vi "General-GetMultValue.vi"(1 "Ultimo Intervalo":dbl, 2 "Primer Intervalo":dbl, 3 "Tiempo Final":dbl, 4 "t":dbl) -> (0 "Out":dbl)   [LabVIEW 2010]
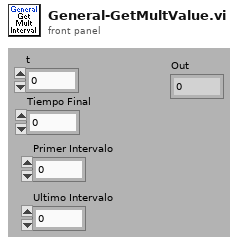
[diagram p1: front panel]
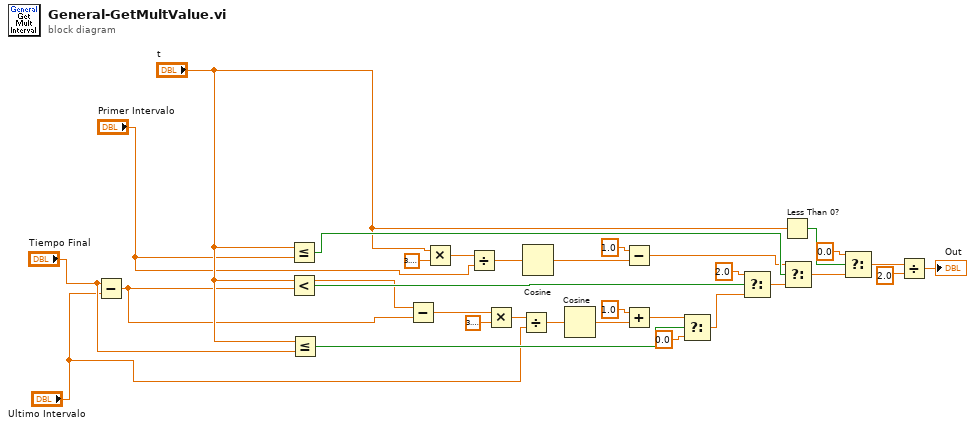
[diagram p0: block diagram]
diagram:
  n1 = Subtract(x="Tiempo Final", y="Ultimo Intervalo") -> (x-y=w3:dbl)
  n2 = Less Or Equal?(x="t", y="Primer Intervalo") -> (x <= y?=w29:bool)
  n3 = Less?(x="t", y=w3) -> (x < y?=w17:bool)
  n4 = Less Or Equal?(x="t", y="Tiempo Final") -> (x <= y?=w10:bool)
  n5 = Subtract(x="t", y=w3) -> (x-y=w14:dbl)
  n6 = Multiply(x="t", y=3.141592653589793) -> (x*y=w28:dbl)
  n7 = Divide(x=w28, y="Primer Intervalo") -> (x/y=w26:dbl)
  n8 = Multiply(x=w14, y=3.141592653589793) -> (x*y=w22:dbl)
  n9 = Divide(x=w22, y="Ultimo Intervalo") -> (x/y=w20:dbl)
  n10 = Cosine(x=w26) -> (cos(x)=w24:dbl)
  n11 = Cosine(x=w20) -> (cos(x)=w18:dbl)
  n12 = Subtract(x=1.0, y=w24) -> (x-y=w13:dbl)
  n13 = Add(x=1.0, y=w18) -> (x+y=w9:dbl)
  n14 = Select(t=w9, s=w10, f=0.0) -> (s? t:f=w7:dbl)
  n15 = Select(t=2.0, s=w17, f=w7) -> (s? t:f=w15:dbl)
  n16 = Less Than 0?(x="t") -> (x < 0?=w31:bool)
  n17 = Select(t=w13, s=w29, f=w15) -> (s? t:f=w23:dbl)
  n18 = Select(t=0.0, s=w31, f=w23) -> (s? t:f=w11:dbl)
  n19 = Divide(x=w11, y=2.0) -> (x/y=→"Out":dbl)
